vi "FT_Open_Device_By_Description.vi"(0 "Device Description":string="TTL232RG-3V3_Application") -> (1 "FT_Status":u32, 2 "Handle":u32)   [LabVIEW 2018]
uses:
  FTD2XX.dll
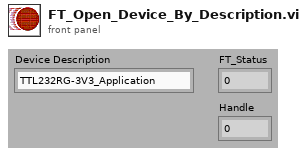
[diagram p1: front panel]
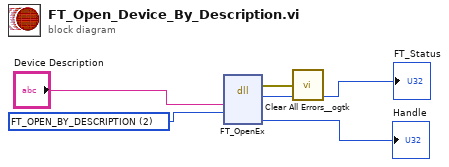
[diagram p0: block diagram]
diagram:
  w2 = u32 2 items=["FT_OPEN_BY_SERIAL_NUMBER"=1, "FT_OPEN_BY_DESCRIPTION"=2, "FT_OPEN_BY_LOCATION"=4] ("Flags")
  n1 = dll-call lib="FTD2XX.dll" fn="FT_OpenEx"("DeviceDescription"="Device Description", "Flags"=w2) -> (error out=w1:errorcluster, "FT_Status"=→"FT_Status":u32, "Handle"=→"Handle":u32)  [unwired: 6 in, 1 out]
  n2 = call <userlib>:"Clear All Errors__ogtk.vi"("Error In"=w1) -> ()  [unwired: 3 in, 1 out]
